vi "timestampToPOSIXtime.vi"(10 "numberToTest":dbl format="%.1f") -> (1 "subtractForPOSIX":dbl format="%.1f", 2 "numberOut":dbl format="%.1f", 3 "looksLikeTimestamp":bool)   [LabVIEW 2022 SP3]
panel:
  in  "timestampEnd":timestamp=timestamp(6216739200 s since 1904-01-01)
  in  "timestampStart":timestamp=timestamp(2650838400 s since 1904-01-01)
  # "If number is in range likely to be timestamp, adjust by POSIX offset"
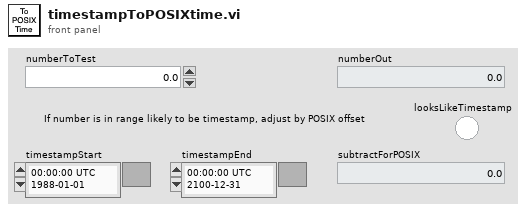
[diagram p1: front panel]
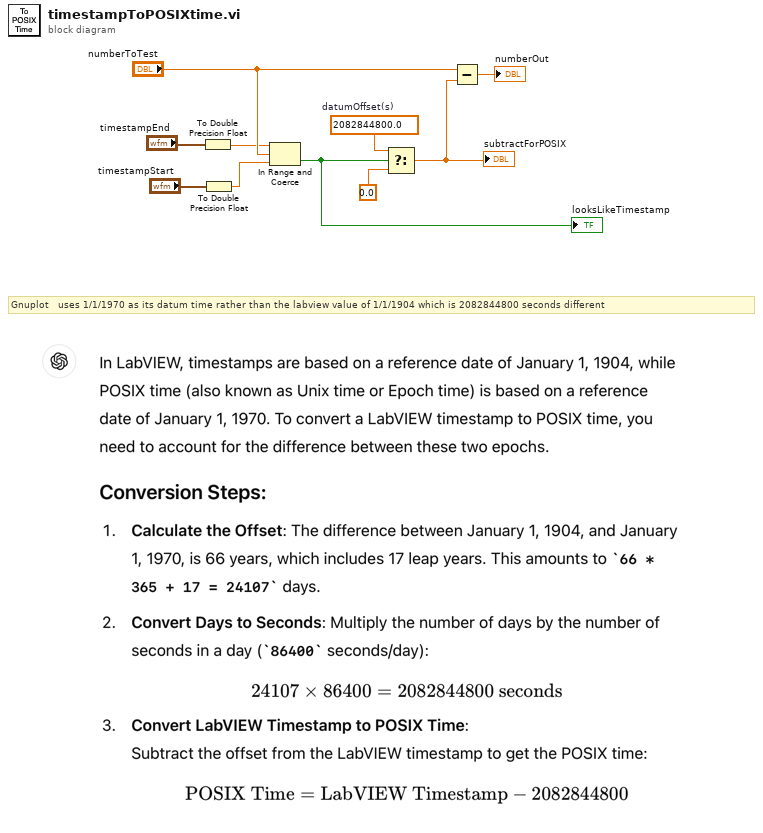
[diagram p0: block diagram]
diagram:
  w9 = 2082844800.0  # datumOffset(s)
  # "Gnuplot   uses 1/1/1970 as its datum time rather than the labview value of 1/1/1904 which is 2082844800 seconds different"
  n1 = To Double Precision Float(number="timestampEnd") -> (double precision float=w3:dbl)
  n2 = To Double Precision Float(number="timestampStart") -> (double precision float=w4:dbl)
  n3 = In Range and Coerce(upper limit=w3, x="numberToTest", lower limit=w4) -> (In Range?=w1:bool)  [unwired: 1 out]
  "looksLikeTimestamp" <- w1
  n4 = Select(t=w9, s=w1, f=0.0) -> (s? t:f=w7:dbl)
  "subtractForPOSIX" <- w7
  n5 = Subtract(x="numberToTest", y=w7) -> (x-y=→"numberOut":dbl)
